vi "BallShear_PackageCheck.vi"(11 "Check":bool) -> (3 "Ready":bool)   [LabVIEW 2013]
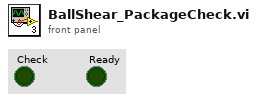
[diagram p1: front panel]
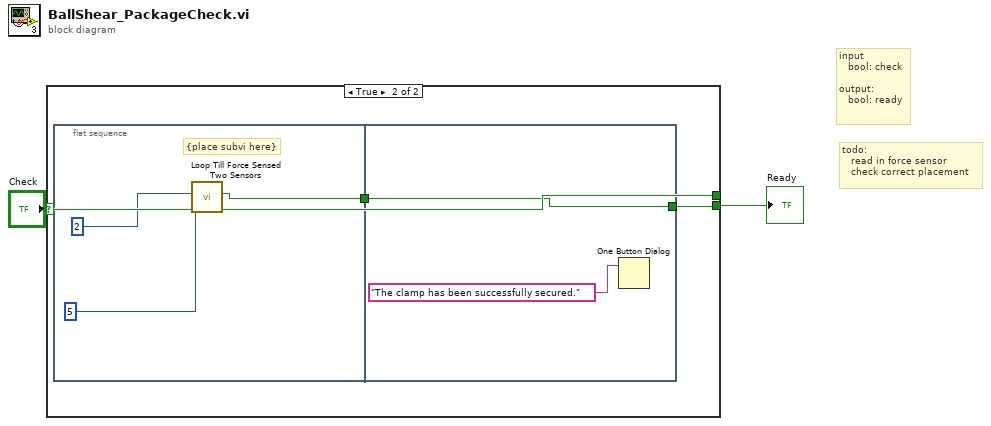
[diagram p0: block diagram]
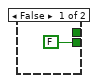
[diagram p2: hidden frame]
diagram:
  # "todo:\n   read in force sensor\n   check correct placement"
  # "input\n   bool: check\n\noutput:\n   bool: ready"
  n1 = case shown="True" "Check" {
    tunnel: "Check" -> [_ _]
    tunnel: [FALSE ("Power") w4] -> w1
    frame False {
    }
    frame True {
      n2 = flat-sequence {
        tunnel: [w6] -> w5
        tunnel: w5 -> [w9]
        tunnel: [w9] -> w4
        frame #0 {
          # "{place subvi here}"
          n3 = call "Loop Till Force Sensed Two Sensors.vi"("Analog Input Pin 2"=u8 5, "Analog Input Pin"=u8 2 ("Force Sensor 1")) -> ("Force Threshhold Reached"=w6:bool)  [unwired: 9 in]
        }
        frame #1 {
          n4 = One Button Dialog(message="The clamp has been successfully secured.") -> ()  [unwired: 1 in, 1 out]
        }
      }
    }
  }
  "Ready" <- w1
